vi "练习2-对数扫频.vi"   [LabVIEW 2021]
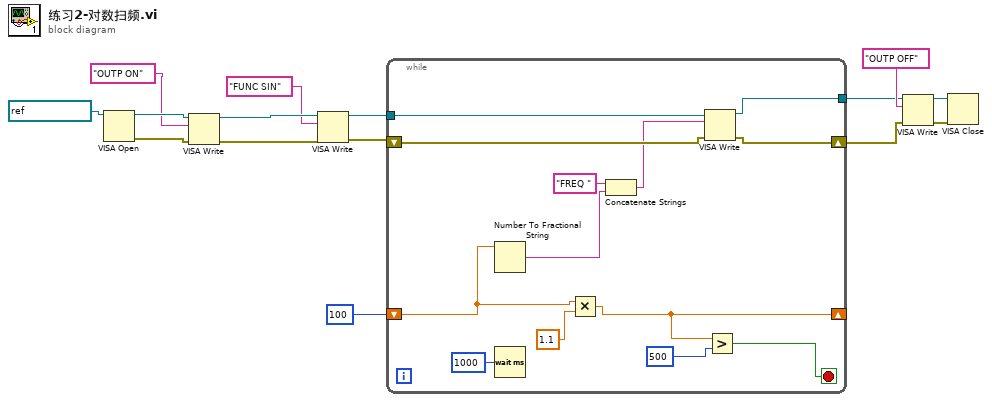
[diagram p0: block diagram]
diagram:
  n1 = VISA Open(VISA resource name=refnum<visa-resource-name> "DG1022U") -> (VISA resource name=w14:refnum<visa-resource-name>, error out=w13:errorcluster)  [unwired: 4 in]
  n2 = VISA Write(VISA resource name=w14, write buffer="OUTP ON", error in (no error)=w13) -> (VISA resource name out=w11:refnum<visa-resource-name>, error out=w9:errorcluster)  [unwired: 1 out]
  n3 = VISA Write(VISA resource name=w11, write buffer="FUNC SIN", error in (no error)=w9) -> (VISA resource name out=w5:refnum<visa-resource-name>, error out=w3:errorcluster)  [unwired: 1 out]
  n4 = while {
    tunnel: w5 -> [w28]
    tunnel: [w27] -> w4
    shift-right: [w25] -> w2
    shift-left: w3 -> [w26]
    shift-right: [w18] -> _
    shift-left: 100 -> [w19]
    stop <- w16 stop-if-true
    n5 = Number To Fractional String(number=w19) -> (F-format string=w22:string)  [unwired: 3 in]
    n6 = Wait (ms)(milliseconds to wait=u32 1000) -> ()  [unwired: 1 out]
    n7 = Multiply(x=w19, y=1.1) -> (x*y=w18:dbl)
    n8 = Concatenate Strings("FREQ " ("string"), w22) -> (w24:string)
    n9 = VISA Write(VISA resource name=w28, write buffer=w24, error in (no error)=w26) -> (VISA resource name out=w27:refnum<visa-resource-name>, error out=w25:errorcluster)  [unwired: 1 out]
    n10 = Greater?(x=w18, y=500) -> (0:w16:bool)
  }
  n11 = VISA Write(VISA resource name=w4, write buffer="OUTP OFF", error in (no error)=w2) -> (VISA resource name out=w7:refnum<visa-resource-name>, error out=w8:errorcluster)  [unwired: 1 out]
  n12 = VISA Close(VISA resource name=w7, error in (no error)=w8) -> ()  [unwired: 1 out]
